vi "Read From Config Spreadsheet File.vi"(4 "delimiter (\\t)":string="\t", 6 "transpose (no:F)":bool, 7 "format (%s)":string="%s", 8 "error in":errorcluster, 11 "file path (dialog if empty)":path) -> (0 "error out":errorcluster, 2 "first row":string[](array[string]), 3 "all rows":string[][](array[string]))   [LabVIEW 2018]
doc: "Reads all lines from a spreadsheet-type delimited configuration file, and converts into a 2D array of strings. Can optionally transpose rows and columns\n\n2008 Bob Hamburger\n2008_04 Added file close, Mike Ashe\nmichael.ashe@imaginatics.net\nCell: 860-961-0876"
panel:
  in  "type (empty)":string[][](array[string])
  # "row\ncolumn"
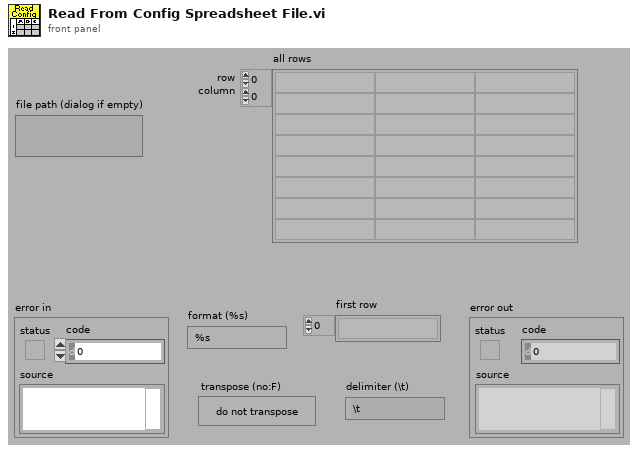
[diagram p1: front panel]
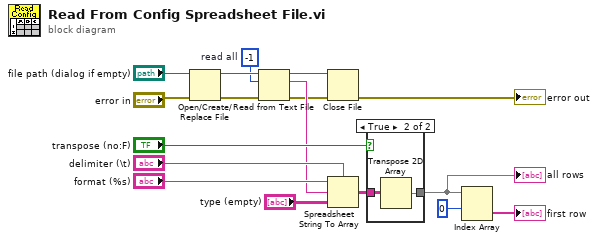
[diagram p0: block diagram]
diagram:
  w6 = -1  # read all
  n1 = Open/Create/Replace File(file path (use dialog)="file path (dialog if empty)", error in="error in") -> (refnum out=w8:refnum<file>, error out=w7:errorcluster)  [unwired: 4 in, 1 out]
  n2 = Read from Text File(file (use dialog)=w8, count=w6, error in=w7) -> (refnum out=w1:refnum<file>, text=w5:string, error out=w3:errorcluster)  [unwired: 1 in, 1 out]
  n3 = Close File(refnum=w1, error in=w3) -> (error out=→"error out":errorcluster)  [unwired: 1 out]
  n4 = Spreadsheet String To Array(delimiter (Tab)="delimiter (\\t)", format string="format (%s)", spreadsheet string=w5, array type (2D Dbl)="type (empty)") -> (array=w12:string[][])
  n5 = case shown="True" "transpose (no:F)" {
    tunnel: w12 -> [w18 w20]
    tunnel: [w18 w19] -> w10
    frame False {
    }
    frame True {
      n6 = Transpose 2D Array(2D array=w20) -> (transposed array=w19:string[][])
    }
  }
  "all rows" <- w10
  n7 = Index Array(array=w10, index (row)=0) -> (element=→"first row":string[])  [unwired: 1 in]
